vi "Configuration - Select First AI Module.vi"(11 "Module Configurations":T1[](array[typedef])) -> (1 "AI Found":bool, 2 "Module Configuration":T1)   [LabVIEW 2017, in "Communications Library.lvlib"]
uses:
  Communications Library.lvlib
  Typedefs/DTACQ Module Configuration--Cluster.ctl
  Typedefs/DTACQ Device Type--Enum.ctl
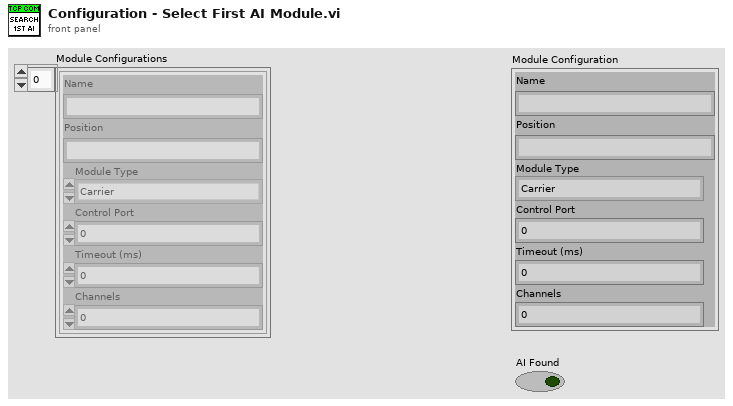
[diagram p1: front panel]
types:
  T1 = typedef "Communications Library.lvlib/DTACQ Module Configuration--Cluster.ctl" = cluster{"Name":string, "Position":string, "Module Type":T2, "Control Port":i32, "Timeout (ms)":i32, "Channels":i32}
  T2 = typedef "Communications Library.lvlib/DTACQ Device Type--Enum.ctl" = enum16{"Carrier", "Analog In Module", "Analog Out Module", "Generic Module"}
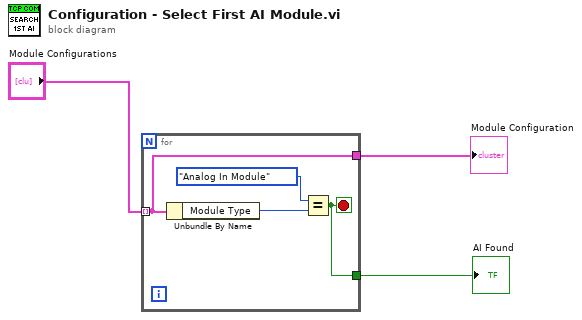
[diagram p0: block diagram]
diagram:
  n1 = for {
    tunnel: "Module Configurations" -> [w5] mode=indexing
    tunnel: [w5] -> w2
    tunnel: [w4] -> w3
    stop <- w4 stop-if-true
    n2 = Unbundle By Name(w5) -> ("Module Type"=w7:T2)
    n3 = Equal?(x=DTACQ_Device_Type--Enum."Analog In Module", y=w7) -> (x = y?=w4:bool)
  }
  "AI Found" <- w3
  "Module Configuration" <- w2
